vi "Determine XML Source Distribution Paths.vi"(10 "Execution Mode":T1, 11 "Targets":enum16{"Linux_x64", "Windows", "All"}(ring)) -> (1 "Targets":string[](array[string]), 2 "Target Paths":string[](array[string]), 3 "Source Paths":string[](array[string]))   [LabVIEW 2026, in "NIVS_CDEW_MetaDataObj.lvclass"]
uses:
  NIVS_CDEW_MetaDataObj.lvclass
  NIVS_CDEW_MetaDataObj.lvclass/NIVS_CDEW_MetaDataObj.ctl
  Types/Execution Modes.ctl
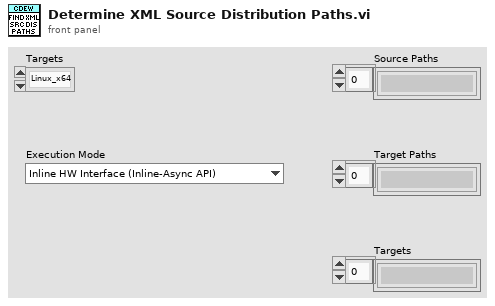
[diagram p1: front panel]
types:
  T1 = typedef "NIVS_CDEW_MetaDataObj.lvclass/Execution Modes.ctl" = enum16{"Inline HW Interface (Inline-Async API)", "Inline HW Interface", "Inline Timing and Sync"}
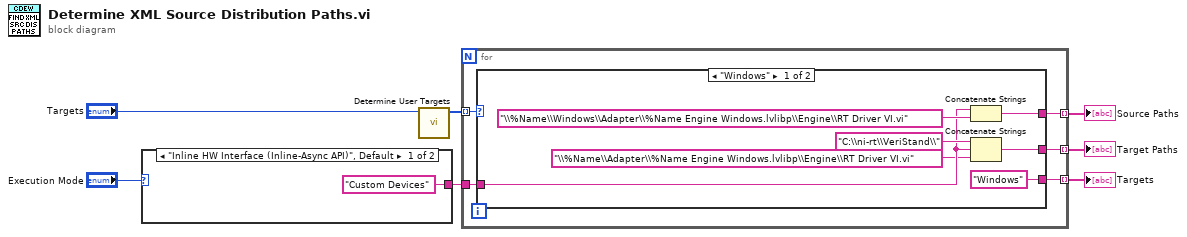
[diagram p0: block diagram]
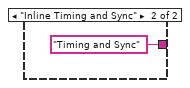
[diagram p2: hidden frame]
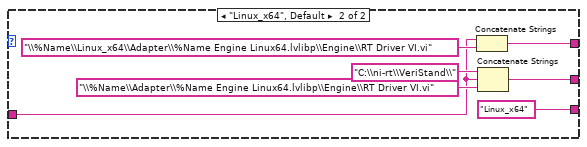
[diagram p3: hidden frame]
diagram:
  n1 = case shown="\"Inline HW Interface (Inline-Async API)\", Default" "Execution Mode" {
    tunnel: ["Custom Devices" "Timing and Sync"] -> w7
    frame "Inline HW Interface (Inline-Async API)", Default {
    }
    frame "Inline Timing and Sync" {
    }
  }
  n2 = call "Determine User Targets.vi"("Targets"="Targets") -> ("User Configured Targets"=w5:enum16{"Linux_x64", "Windows", "All"}[])  [unwired: 10 in]
  n3 = for {
    tunnel: [w14] -> w1 mode=indexing
    tunnel: [w13] -> w2 mode=indexing
    tunnel: [w12] -> w3 mode=indexing
    tunnel: w5 -> [w11] mode=indexing
    tunnel: w7 -> [w10]
    n4 = case shown="\"Windows\"" w11 {
      tunnel: [w17 w25] -> w14
      tunnel: [w19 w26] -> w13
      tunnel: ["Windows" ("Tag Data") "Linux_x64" ("Tag Data")] -> w12
      tunnel: w10 -> [w16 w22]
      frame "Windows" {
        n5 = Concatenate Strings(w16, "\\%Name\\Windows\\Adapter\\%Name Engine Windows.lvlibp\\Engine\\RT Driver VI.vi" ("Tag Data")) -> (w19:string)
        n6 = Concatenate Strings("C:\\ni-rt\\VeriStand\\" ("Tag Data"), w16, "\\%Name\\Adapter\\%Name Engine Windows.lvlibp\\Engine\\RT Driver VI.vi" ("Tag Data")) -> (w17:string)
      }
      frame "Linux_x64", Default {
        n7 = Concatenate Strings(w22, "\\%Name\\Linux_x64\\Adapter\\%Name Engine Linux64.lvlibp\\Engine\\RT Driver VI.vi" ("Tag Data")) -> (w26:string)
        n8 = Concatenate Strings("C:\\ni-rt\\VeriStand\\" ("Tag Data"), w22, "\\%Name\\Adapter\\%Name Engine Linux64.lvlibp\\Engine\\RT Driver VI.vi" ("Tag Data")) -> (w25:string)
      }
    }
  }
  "Targets" <- w3
  "Source Paths" <- w2
  "Target Paths" <- w1
